vi "Update Temperature.vi"(8 "error in (no error)":errorcluster, 10 "Temperature":dbl, 11 "Top Level in":refnum<class "Top Level.lvclass">) -> (0 "error out":errorcluster, 3 "Top Level out":refnum<class "Top Level.lvclass">)   [LabVIEW 2021, in "Top Level.lvlib" / "Top Level.lvclass"]
uses:
  Top Level.lvclass
  Top Level.lvclass/Top Level.ctl
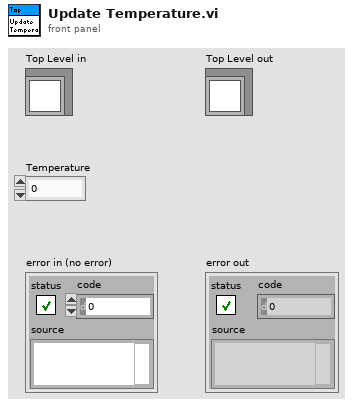
[diagram p1: front panel]
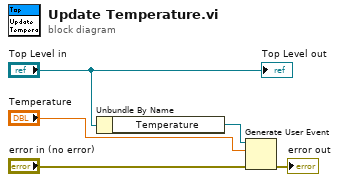
[diagram p0: block diagram]
diagram:
  n1 = Unbundle By Name("Top Level in") -> ("Temperature"=w4:refnum<user-event>)
  n2 = Generate User Event(user event=w4, event data cluster="Temperature", error in="error in (no error)") -> (error out=→"error out":errorcluster)  [unwired: 1 in, 1 out]
  "Top Level out" <- "Top Level in"
